vi "isPath.vi"(7 "path Current VI":path, 8 "error in TCP":errorcluster, 10 "string Path in":string, 11 "connection ID in":refnum<k5>) -> (0 "error out TCP":errorcluster, 1 "Path is Ok?":bool, 2 "absolute path":path, 3 "connection ID out":refnum<k5>)   [LabVIEW 2010]
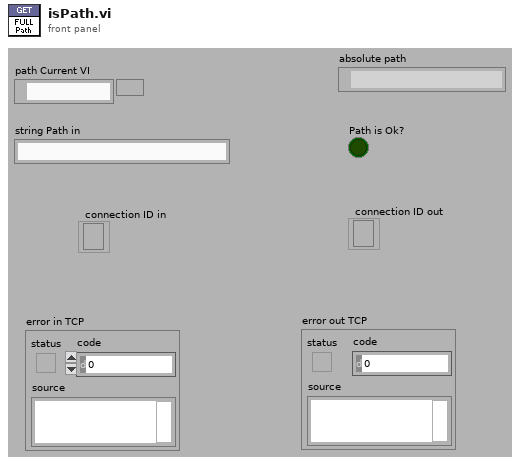
[diagram p1: front panel]
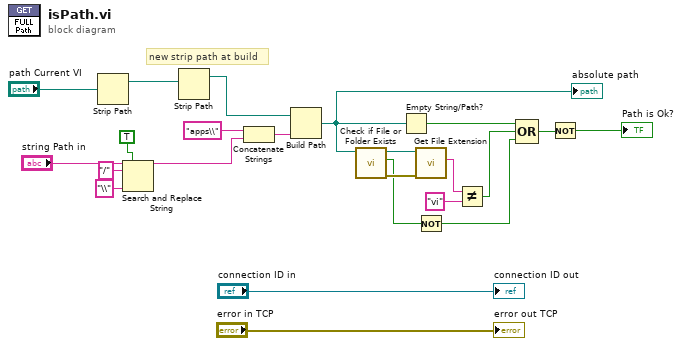
[diagram p0: block diagram]
diagram:
  # "new strip path at build"
  n1 = Strip Path(path="path Current VI") -> (stripped path=w2:path)  [unwired: 1 out]
  n2 = Search and Replace String(replace all?=TRUE ("replace all? (F)"), input string="string Path in", search string="/", replace string="\\" ("replace string (\"\")")) -> (result string=w6:string)  [unwired: 1 in, 6 out]
  n3 = Strip Path(path=w2) -> (stripped path=w1:path)  [unwired: 1 out]
  n4 = Concatenate Strings("apps\\" ("string"), w6) -> (w23:string)
  n5 = Build Path(base path=w1, name or relative path=w23) -> (appended path=w14:path)
  "absolute path" <- w14
  n6 = call <vilib>:"Check if File or Folder Exists.vi"("path"=w14) -> ("error out"=w20:errorcluster, "file or folder exists?"=w16:bool, "dup path"=w21:path)  [unwired: 1 in, 7 out]
  n7 = Empty String/Path?(string/path=w14) -> (empty?=w18:bool)
  n8 = call <vilib>:"Get File Extension.vi"("error in (no error)"=w20, "file"=w21) -> ("lowercase file extension"=w3:string)  [unwired: 9 out]
  n9 = Not(x=w16) -> (.not. x?=w15:bool)
  n10 = Not Equal?(x=w3, y="vi") -> (x != y?=w17:bool)
  n11 = Compound Arithmetic op=OR(w18, w17, w15) -> (w5:bool)
  n12 = Not(x=w5) -> (.not. x?=→"Path is Ok?":bool)
  "connection ID out" <- "connection ID in"
  "error out TCP" <- "error in TCP"
